vi "Xeryon Axis receive command.vi"(0 "queue out":refnum<queue>) -> (1 "Type":enum16{"Message", "Timeout"}(ring), 2 "Serial Message":T1={"Command"=enum."Exit", "Data to send"=""}, 3 "Send feedback":bool)   [LabVIEW 2014]
uses:
  Xeryon Axis command.ctl
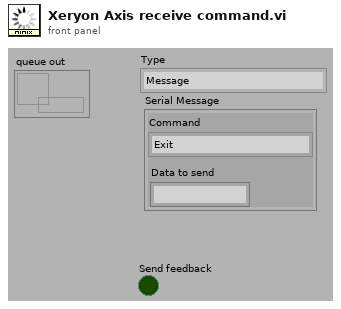
[diagram p1: front panel]
types:
  T1 = typedef "Xeryon Axis command.ctl" = cluster{"Command":enum16{"Reset", "Zero output", "Go home", "Find index", "Scan -X", "Scan +X", "Scan Stop", "Step -X", "Step +X", "Set DPOS", "Stop", "Continue", "Desired speed", "Apply settings file", "Exit", "Reset encoder", "Recover", "Save"}, "Data to send":string}
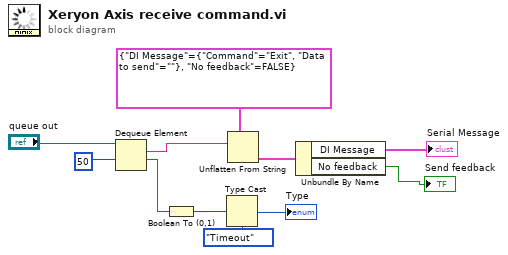
[diagram p0: block diagram]
diagram:
  n1 = Dequeue Element(queue="queue out", timeout in ms (-1)=50) -> (element=w3:string, timed out?=w2:bool)  [unwired: 1 in, 2 out]
  n2 = Boolean To (0,1)(Boolean=w2) -> (0, 1=w10:i16)
  n3 = Type Cast(type=enum16{"Message", "Timeout"}."Timeout" ("Command"), x=w10) -> (*(type *) &x=→"Type":enum16{"Message", "Timeout"})
  n4 = Unflatten From String(type=cluster{"DI Message":T1, "No feedback":bool} {"DI Message"={"Command"=enum."Exit", "Data to send"=""}, "No feedback"=FALSE} ("output cluster"), binary string=w3) -> (value=w7:cluster{"DI Message":T1, "No feedback":bool})  [unwired: 1 in, 4 out]
  n5 = Unbundle By Name(w7) -> ("DI Message"=→"Serial Message":T1, "No feedback"=→"Send feedback":bool)
